vi "tt-构建扇形ROI-A型式.vi"(5 "R_ROI小圆半径":i32=225, 6 "开启调试显示":bool, 7 "钩端向上部偏移量":dbl=110.0, 8 "error in (no error)":errorcluster, 9 "镜像产品角度":dbl=45.0, 10 "扇形半张角":dbl=30.0 format="%#_13g", 11 "ImageSrc":T3(plugin-control)) -> (0 "error out":errorcluster, 1 "anROI":T2 {"Contours"."Type" items=["No Selection", "Point", "Line", "Rectangle", "Oval", "Polygon", "Freehand Region", "Annulus", "Unused2", "Unused3", "Broken Line", "Freehand Line", "Rotated Rectangle"]}, 2 "输出RECT":T1 {"End Angle" min=-90.0 max=90.0 step=1.0 format="%.2f"; "Start Angle" min=-90.0 max=90.0 step=1.0 format="%.2f"; "Center X" scale=0.0..1024.0}, 3 "ImgOut":T3(plugin-control))   [LabVIEW 2018]
uses:
  <vilib>/vision/NI_Vision_Development_Module.lvlib
panel:
  in  "Annulus":T1={"Center X"=0, "Center Y"=0, "Inner Radius"=27, "Outer Radius"=107, "Start Angle"=0.0, "End Angle"=0.0} {"End Angle" min=-90.0 max=90.0 step=1.0 format="%.2f"; "Start Angle" min=-90.0 max=90.0 step=1.0 format="%.2f"; "Center X" scale=0.0..1024.0}
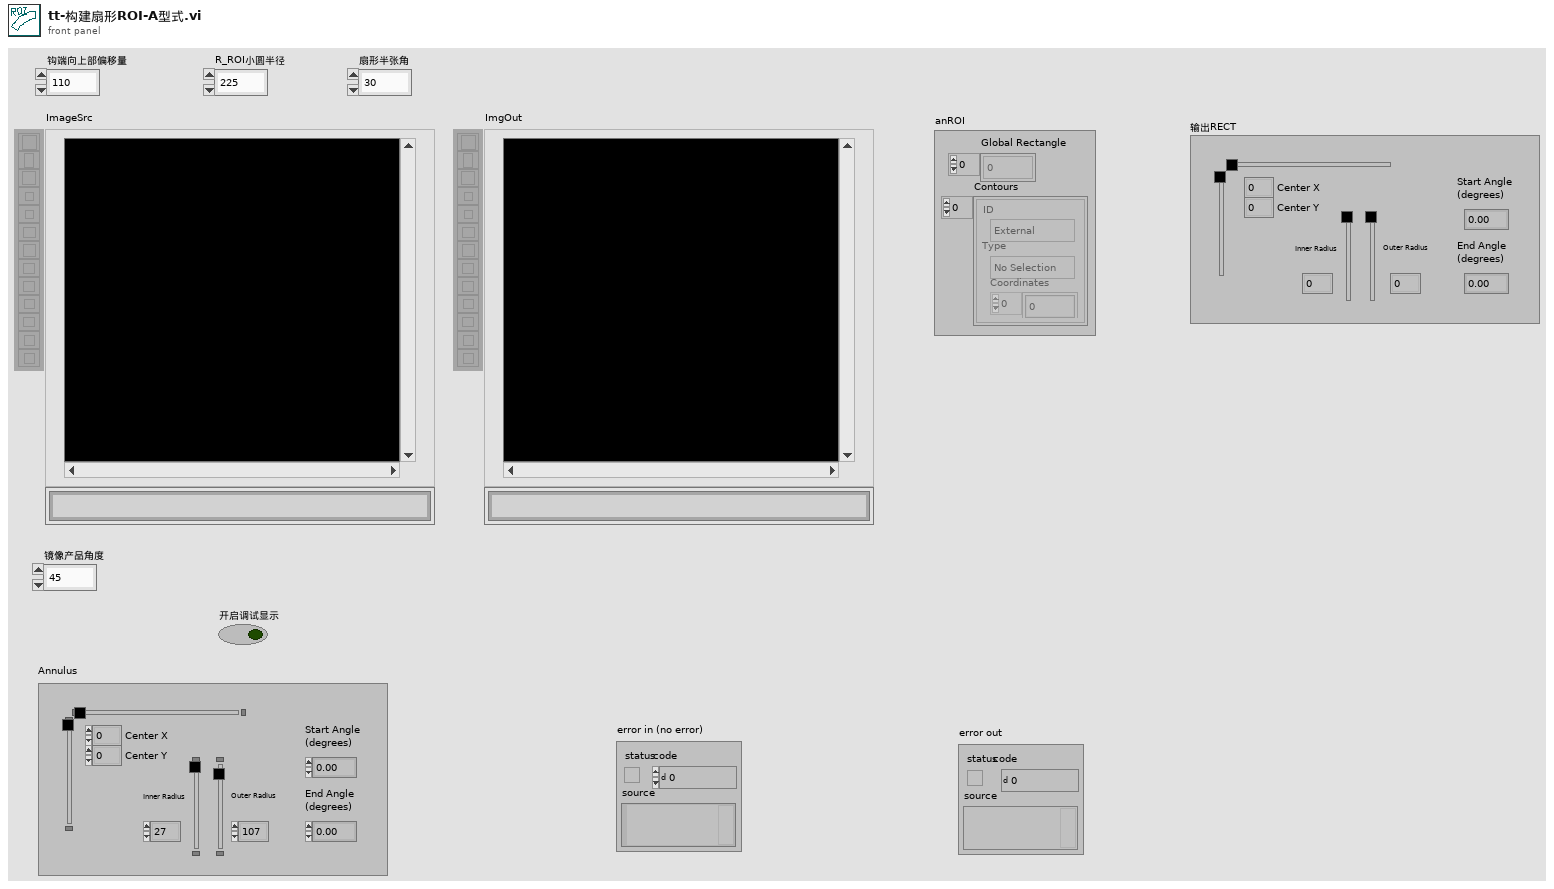
[diagram p1: front panel]
types:
  T1 = typedef "IMAQ Circle" = cluster{"Center X":i32, "Center Y":i32, "Inner Radius":i32, "Outer Radius":i32, "Start Angle":dbl, "End Angle":dbl}
  T2 = typedef "ROI Descriptor" = cluster{"Global Rectangle":i32[], "Contours":cluster{"ID":enum32{"External", "Internal"}, "Type":u32, "Coordinates":i32[]}[]}
  T3 = typedef "IMAQ Image.ctl" = refnum<image>
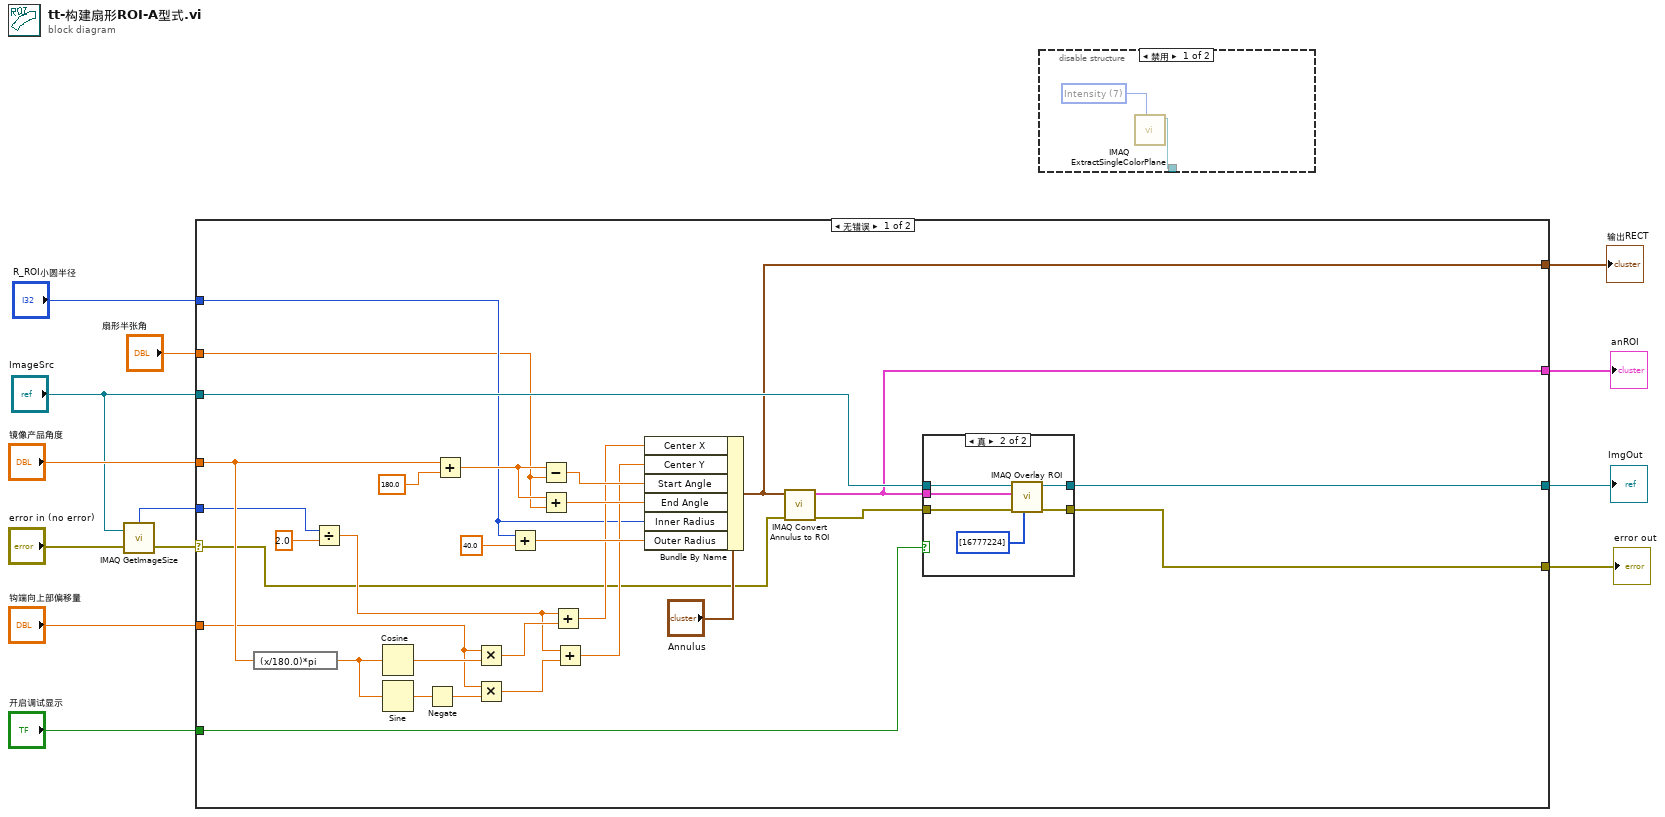
[diagram p0: block diagram]
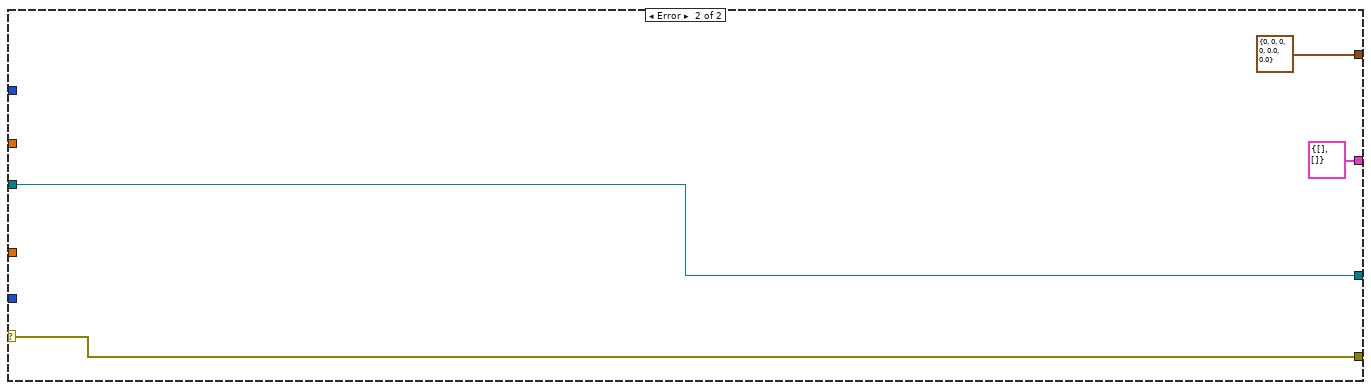
[diagram p4: hidden frame]
diagram:
  n1 = call "IMAQ GetImageSize"("Image"="ImageSrc", "error in (no error)"="error in (no error)") -> ("X Resolution"=w4:i32, "error out"=w11:errorcluster)  [unwired: 2 in, 1 out]
  n2 = case shown="无错误" w11 {
    selector: w11 -> [w20 w54]
    tunnel: "镜像产品角度" -> [w35 _]
    tunnel: "ImageSrc" -> [w23 w55]
    tunnel: "钩端向上部偏移量" -> [w30 _]
    tunnel: [w24 w55] -> w9
    tunnel: [w22 w54] -> w8
    tunnel: "开启调试显示" -> [w19 _]
    tunnel: [w18 T2 {"Global Rectangle"=[], "Contours"=[]} ("ROI Descriptor")] -> w6
    tunnel: w4 -> [w17 _]
    tunnel: "R_ROI小圆半径" -> [w16 _]
    tunnel: "扇形半张角" -> [w15 _]
    tunnel: [w14 T1 {"Center X"=0, "Center Y"=0, "Inner Radius"=0, "Outer Radius"=0, "Start Angle"=0.0, "End Angle"=0.0} ("Annulus")] -> w1
    frame No Error {
      n3 = expression code="(x/180.0)*pi" ("角度转换至弧度")(w35) -> (w33:dbl)
      n4 = Divide(x=w17, y=2.0) -> (x/y=w26:dbl)
      n5 = Cosine(x=w33) -> (cos(x)=w32:dbl)
      n6 = Sine(x=w33) -> (sin(x)=w34:dbl)
      n7 = Negate(x=w34) -> (-x=w31:dbl)
      n8 = Add(x=w35, y=180.0) -> (x+y=w41:dbl)
      n9 = Multiply(x=w30, y=w32) -> (x*y=w29:dbl)
      n10 = Multiply(x=w30, y=w31) -> (x*y=w27:dbl)
      n11 = Add(x=w16, y=40.0) -> (x+y=w36:dbl)
      n12 = Subtract(x=w41, y=w15) -> (x-y=w40:dbl)
      n13 = Add(x=w41, y=w15) -> (x+y=w39:dbl)
      n14 = Add(x=w26, y=w29) -> (x+y=w28:dbl)
      n15 = Add(x=w26, y=w27) -> (x+y=w25:dbl)
      n16 = Bundle By Name(cluster="Annulus", "Center X"=w28, "Center Y"=w25, "Start Angle"=w40, "End Angle"=w39, "Inner Radius"=w16, "Outer Radius"=w36) -> (w14:T1)
      n17 = call "IMAQ Convert Annulus to ROI"("error in (no error)"=w20, "Annulus"=w14) -> ("error out"=w21:errorcluster, "ROI Descriptor"=w18:T2)  [unwired: 7 in]
      n18 = case shown="真" w19 {
        tunnel: [w44 w50] -> w24
        tunnel: w18 -> [_ w49]
        tunnel: w23 -> [w44 w48]
        tunnel: [w45 w47] -> w22
        tunnel: w21 -> [w45 w46]
        frame False {
        }
        frame True {
          n19 = call "IMAQ Overlay ROI"("Colors (Green)"=u32[] [16777224], "error in (no error)"=w46, "ROI Descriptor"=w49, "Image"=w48) -> ("error out"=w47:errorcluster, "Image Out"=w50:T3)  [unwired: 6 in]
        }
      }
    }
    frame Error {
    }
  }
  "ImgOut" <- w9
  "error out" <- w8
  "anROI" <- w6
  "输出RECT" <- w1
  n20 = disable-structure shown="禁用" {
    disable-tunnel: [w56 _] -> _
    frame Disabled {
      w57 = 7 items=["Red", "Green", "Blue", "Hue", "Saturation", "Luminance", "Value", "Intensity"] ("Color Plane")
      n21 = call "IMAQ ExtractSingleColorPlane"("Color Plane"=w57) -> ("Image Dst Out"=w56:T3)  [unwired: 9 in, 1 out]
    }
    frame Enabled {
    }
  }
